vi "initialize can fd.vi"(8 "error in (no error)":errorcluster, 10 "bitrate":T1={"clock frequency"=enum."CLOCK_80MHz", "nominal bitrate"={"bitrate prescaler"=2, "time segment 1"=63, "time segment 2"=16, "sync jump width"=16}, "data bitrate"={"bitrate prescaler"=2, "time segment 1"=15, "time segment 2"=4, "sync jump width"=4}}, 11 "channel":u16 format="%x") -> (0 "error out":errorcluster)   [LabVIEW 2024, in "atsj peakcan basic.lvlib"]
doc: "Initializes an FD-capable PeakCAN <b>channel</b>."
uses:
  atsj peakcan basic.lvlib
  support/x64/PCANBasic.dll
  clock frequency.ctl
  can fd bitrate parameters.ctl
  can fd bitrate.ctl
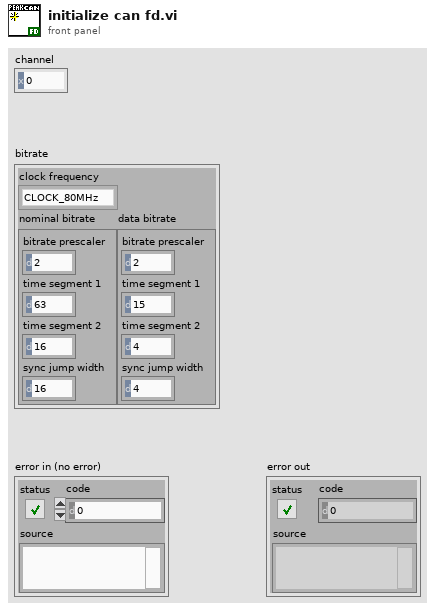
[diagram p1: front panel]
types:
  T1 = typedef "atsj peakcan basic.lvlib/can fd bitrate.ctl" = cluster{"clock frequency":T2, "nominal bitrate":T3, "data bitrate":T3}
  T2 = typedef "atsj peakcan basic.lvlib/clock frequency.ctl" = enum16{"CLOCK_80MHz", "CLOCK_60MHz", "CLOCK_40MHz", "CLOCK_30MHz", "CLOCK_24MHz", "CLOCK_20MHz"}
  T3 = typedef "atsj peakcan basic.lvlib/can fd bitrate parameters.ctl" = cluster{"bitrate prescaler":u16, "time segment 1":u16, "time segment 2":u16, "sync jump width":u16}
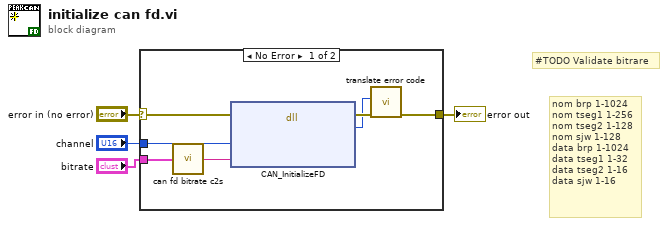
[diagram p0: block diagram]
diagram:
  # "nom brp 1-1024\nnom tseg1 1-256\nnom tseg2 1-128\nnom sjw 1-128\ndata brp 1-1024\ndata tseg1 1-32\ndata tseg2 1-16\ndata sjw 1-16"
  # "#TODO Validate bitrare"
  n1 = case shown="No Error" "error in (no error)" {
    selector: "error in (no error)" -> [w11 w12]
    tunnel: [w6 w12] -> w3
    tunnel: "channel" -> [w10 _]
    tunnel: "bitrate" -> [w9 _]
    frame No Error {
      n2 = call "can fd bitrate c2s.vi"("bitrate"=w9) -> ("bitrate string"=w8:string)
      n3 = dll-call lib="C:/atsj/plateau/atsj-peakcan-basic-for-labview/src/support/x64/PCANBasic.dll" fn="CAN_InitializeFD" ("initialize fd")(error in=w11, "Channel"=w10, "BitrateFD"=w8) -> (error out=w7:errorcluster, "Status"=w5:u32)  [unwired: 4 in, 1 out]
      n4 = call "translate error code.vi"("error in (no error)"=w7, "error code"=w5) -> ("error out"=w6:errorcluster)  [unwired: 9 in]
    }
    frame Error {
    }
  }
  "error out" <- w3
